vi "Cal Interpolation.vi"() -> ()   [LabVIEW 2018]
doc: "This example shows the operation of the 1D interpolation VI using three selectable test sets."
uses:
  <vilib>/Utility/file.llb/Read From Spreadsheet File (DBL).vi
  <vilib>/gmath/NI_Gmath.lvlib
panel:
  out "size(s)":i32[](array[numeric])=[295001, 2]
  in  "index (row)":i32=1
  in  "stop":bool
  in  "Tab Control":enum32{"Graph", "Data"}(tab)
  out "1D Interpolation Graph":cluster{"yi":dbl[], "ramp data":dbl[]}[](graph)=[{"yi"=[50000000.0, 100000000.0, 150000000.0, 200000000.0, 250000000.0, 300000000.0, 350000000.0, 400000000.0, 450000000.0, 500000000.0, 550000000.0, 600000000.0, 650000000.0, 700000000.0, 750000000.0, 800000000.0, 850000000.0, 900000000.0, 950000000.0, 1000000000.0, 1050000000.0, 1100000000.0, 1150000000.0, 1200000000.0, 1250000000.0, 1300000000.0, 1350000000.0, 1400000000.0, 1450000000.0, 1500000000.0, 1550000000.0, 1600000000.0, 1650000000.0, 1700000000.0, 1750000000.0, 1800000000.0, 1850000000.0, 1900000000.0, 1950000000.0, 2000000000.0, 2050000000.0, 2100000000.0, 2150000000.0, 2200000000.0, 2250000000.0, 2300000000.0, 2350000000.0, 2400000000.0, 2450000000.0, 2500000000.0, 2550000000.0, 2600000000.0, 2650000000.0, 2700000000.0, 2750000000.0, 2800000000.0, 2850000000.0, 2900000000.0, 2950000000.0, 3000000000.0], "ramp data"=[-0.08, -0.16, -0.21, -0.23, -0.24, -0.28, -0.3, -0.34, -0.33, -0.31, -0.38, -0.37, -0.42, -0.39, -0.48, -0.41, -0.45, -0.41, -0.46, -0.48, -0.53, -0.57, -0.58, -0.65, -0.6, -0.71, -0.66, -0.77, -0.68, -0.78, -0.76, -0.88, -0.81, -0.83, -0.87, -0.83, -0.97, -0.81, -0.92, -0.79, -1.11, -0.76, -0.94, -0.98, -1.08, -0.9, -0.89, -1.14, -1.07, -1.25, -0.93, -1.25, -0.97, -1.38, -1.03, -1.17, -1.06, -1.21, -1.13, -0.98]}, {"yi"=array[295001 elements], "ramp data"=array[295001 elements]}]
  out "Interpolated Data":dbl[][](array[numeric])
  out "Original Data":dbl[][](array[numeric])=[[50000000.0, -0.08], [100000000.0, -0.16], [150000000.0, -0.21], [200000000.0, -0.23], [250000000.0, -0.24], [300000000.0, -0.28], [350000000.0, -0.3], [400000000.0, -0.34], [450000000.0, -0.33], [500000000.0, -0.31], [550000000.0, -0.38], [600000000.0, -0.37], [650000000.0, -0.42], [700000000.0, -0.39], [750000000.0, -0.48], [800000000.0, -0.41], [850000000.0, -0.45], [900000000.0, -0.41], [950000000.0, -0.46], [1000000000.0, -0.48], [1050000000.0, -0.53], [1100000000.0, -0.57], [1150000000.0, -0.58], [1200000000.0, -0.65], [1250000000.0, -0.6], [1300000000.0, -0.71], [1350000000.0, -0.66], [1400000000.0, -0.77], [1450000000.0, -0.68], [1500000000.0, -0.78], [1550000000.0, -0.76], [1600000000.0, -0.88], [1650000000.0, -0.81], [1700000000.0, -0.83], [1750000000.0, -0.87], [1800000000.0, -0.83], [1850000000.0, -0.97], [1900000000.0, -0.81], [1950000000.0, -0.92], [2000000000.0, -0.79], [2050000000.0, -1.11], [2100000000.0, -0.76], [2150000000.0, -0.94], [2200000000.0, -0.98], [2250000000.0, -1.08], [2300000000.0, -0.9], [2350000000.0, -0.89], [2400000000.0, -1.14], [2450000000.0, -1.07], [2500000000.0, -1.25], [2550000000.0, -0.93], [2600000000.0, -1.25], [2650000000.0, -0.97], [2700000000.0, -1.38], [2750000000.0, -1.03], [2800000000.0, -1.17], [2850000000.0, -1.06], [2900000000.0, -1.21], [2950000000.0, -1.13], [3000000000.0, -0.98]]
  in  "Method":i32(ring)=1 items=["nearest", "linear", "spline", "cubic Hermite", "Lagrange"]
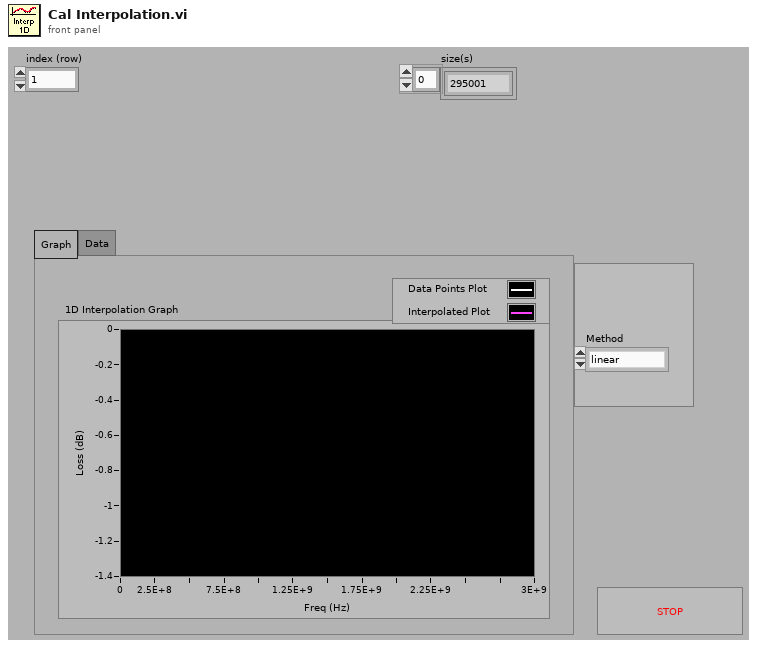
[diagram p1: front panel]
types:
  T1 = cluster{"starting value":dbl, "increment":dbl, "final value":dbl}
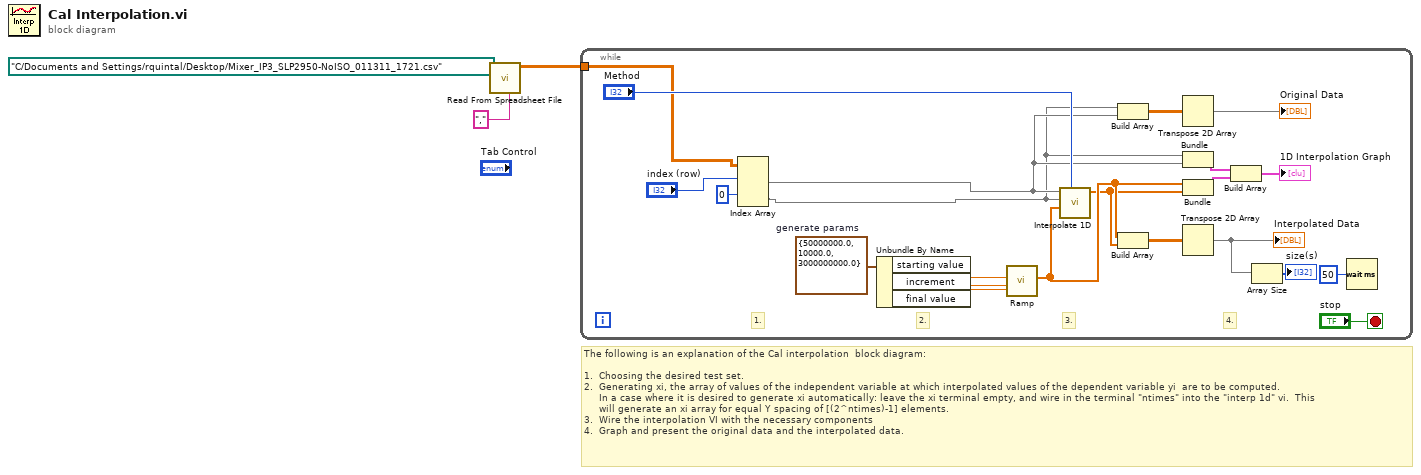
[diagram p0: block diagram]
diagram:
  # "The following is an explanation of the Cal interpolation  block diagram:\n\n1.  Choosing the desired test set.\n2.  Generating xi, the array of values of the independent variable at which interpolated values of the dependent variable yi  are to be computed. \n     In a case where it is desired to generate xi automatically: leave the xi terminal empty, and wire in the terminal \"ntimes\" into the \"interp 1d\" vi.  This\n     will generate an xi array for equal Y spacing of [(2^ntimes)-1] elements.\n3.  Wire the interpolation VI with the necessary components\n4.  Graph and present the original data and the interpolated data."
  n1 = call-poly <vilib>:"Read From Spreadsheet File.vi"("delimiter (\\t)"="," ("delimiter (\\t)"), "file path (dialog if empty)"=path "C:/Documents and Settings/rquintal/Desktop/Mixer_IP3_SLP2950-NoISO_011311_1721.csv") -> ("all rows"=w3:dbl[][])  [unwired: 5 in, 4 out]
  n2 = while {
    tunnel: w3 -> [w11]
    stop <- "stop" stop-if-true
    w6 = T1 {"starting value"=50000000.0, "increment"=10000.0, "final value"=3000000000.0}  # generate params
    # "4."
    # "3."
    # "2."
    # "1."
    n3 = Index Array(array=w11, index (row) #1="index (row)", index (row) #2=0 ("index (row)")) -> (element #1=w10:dbl[], element #2=w9:dbl[])  [unwired: 2 in]
    n4 = Unbundle By Name(w6) -> ("starting value"=w20:dbl, "increment"=w19:dbl, "final value"=w18:dbl)
    n5 = call "Ramp.vi"("# of Samples"=w18, "Start"=w19, "Stop"=w20) -> ("Output"=w14:dbl[])  [unwired: 8 in]
    n6 = call <vilib>:"Interpolate 1D.vi"("method"="Method", "xi"=w14, "X"=w9, "Y"=w10) -> ("yi"=w13:dbl[])  [unwired: 5 in, 2 out]
    n7 = Build Array(w9, w10) -> (w17:dbl[][])
    n8 = Build Array(w14, w13) -> (w15:dbl[][])
    n9 = Transpose 2D Array(2D array=w17) -> (transposed array=→"Original Data":dbl[][])
    n10 = Bundle("all rows"=w9, "all rows"=w10) -> (w22:cluster{"all rows":dbl[], "all rows":dbl[]})  [unwired: 1 in]
    n11 = Bundle("Output"=w14, "yi"=w13) -> (w23:cluster{"Output":dbl[], "yi":dbl[]})  [unwired: 1 in]
    n12 = Transpose 2D Array(2D array=w15) -> (transposed array=w5:dbl[][])
    "Interpolated Data" <- w5
    n13 = Build Array(w22, w23) -> (→"1D Interpolation Graph":cluster{"Output":dbl[], "yi":dbl[]}[])
    n14 = Array Size(array=w5) -> (size(s)=→"size(s)":i32[])
    n15 = Wait (ms)(milliseconds to wait=u32 50) -> ()  [unwired: 1 out]
  }
